vi "Set Report Footer Text.vi"(0 "report in":refnum<class "NI_Standard Report.lvclass">, 5 "left footer text":string, 7 "center footer text":string, 9 "right footer text":string, 11 "error in (no error)":errorcluster, 12 "HTML footer size":enum16{"H1", "H2", "H3", "H4", "H5", "H6", "H7"}(ring)=enum."H3") -> (4 "report out":refnum<class "NI_Standard Report.lvclass">, 15 "error out":errorcluster)   [LabVIEW 2015, in "NI_Standard Report.lvclass"]
doc: "Sets the text of the report footer."
uses:
  <vilib>/Utility/NIReport.llb/Standard Report/NI_Standard Report.lvclass
  <vilib>/Utility/NIReport.llb/Standard Report/NI_Standard Report.lvclass/NI_Standard Report.ctl
  <vilib>/Utility/NIReport.llb/NI_ReportGenerationCore.lvlib
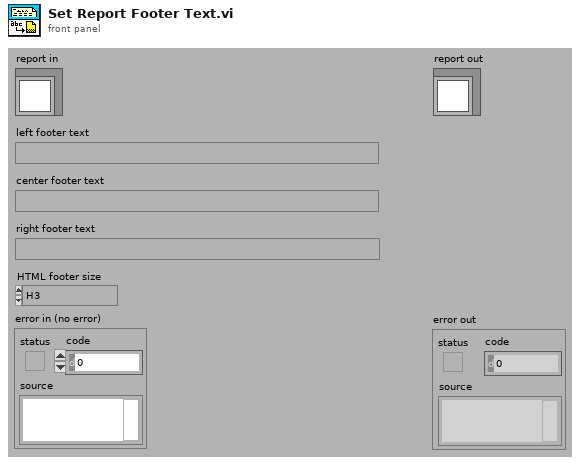
[diagram p1: front panel]
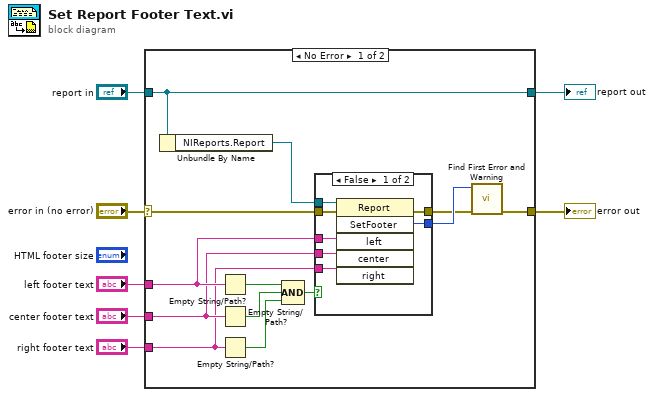
[diagram p0: block diagram]
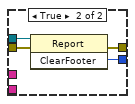
[diagram p2: hidden frame]
diagram:
  n1 = case shown="No Error" "error in (no error)" {
    selector: "error in (no error)" -> [w9 w33]
    tunnel: [w8 w33] -> w6
    tunnel: [w10 w32] -> w4
    tunnel: "report in" -> [w10 w32]
    tunnel: "left footer text" -> [w13 _]
    tunnel: "center footer text" -> [w12 _]
    tunnel: "right footer text" -> [w11 _]
    frame No Error {
      n2 = Unbundle By Name(w10) -> ("NIReports.Report"=w14:refnum<k7>)
      n3 = Empty String/Path?(string/path=w13) -> (empty?=w18:bool)
      n4 = Empty String/Path?(string/path=w12) -> (empty?=w19:bool)
      n5 = Empty String/Path?(string/path=w11) -> (empty?=w20:bool)
      n6 = Compound Arithmetic op=AND(w18, w19, w20) -> (w17:bool)
      n7 = case shown="False" w17 {
        tunnel: w13 -> [w27 _]
        tunnel: w12 -> [w26 _]
        tunnel: w11 -> [w25 _]
        tunnel: [w24 w28] -> w16
        tunnel: [w23 w29] -> w15
        tunnel: w9 -> [w22 w30]
        tunnel: w14 -> [w21 w31]
        frame False {
          n8 = invoke class="Report" method="SetFooter"(reference=w21, error in=w22, "left"=w27, "center"=w26, "right"=w25) -> (error out=w23:errorcluster, "SetFooter"=w24:i32)  [unwired: 1 in, 4 out]
        }
        frame True {
          n9 = invoke class="Report" method="ClearFooter"(reference=w31, error in=w30) -> (error out=w29:errorcluster, "ClearFooter"=w28:i32)  [unwired: 1 in, 1 out]
        }
      }
      n10 = call <vilib>:"Find First Error and Warning.vi"("error in (no error)"=w15, "error code"=w16) -> ("error out"=w8:errorcluster)  [unwired: 1 in, 4 out]
    }
    frame Error {
    }
  }
  "error out" <- w6
  "report out" <- w4
